vi "gamma_0__v1.vi"(10 "ƒÀ[0]":ext, 11 "ƒ¿[0]":ext) -> (3 "ƒÁ[0]":ext)   [LabVIEW 2020]
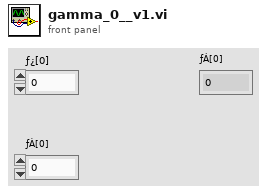
[diagram p1: front panel]
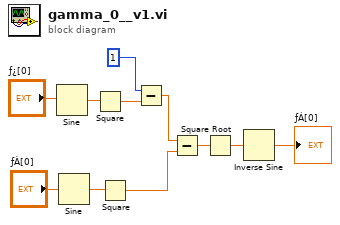
[diagram p0: block diagram]
diagram:
  n1 = Sine(x="ƒ¿[0]") -> (sin(x)=w9:ext)
  n2 = Sine(x="ƒÀ[0]") -> (sin(x)=w8:ext)
  n3 = Square(x=w9) -> (x^2=w7:ext)
  n4 = Square(x=w8) -> (x^2=w4:ext)
  n5 = Subtract(x=1, y=w7) -> (x-y=w5:ext)
  n6 = Subtract(x=w5, y=w4) -> (x-y=w3:ext)
  n7 = Square Root(x=w3) -> (sqrt(x)=w2:ext)
  n8 = Inverse Sine(1:w2) -> (0:→"ƒÁ[0]":ext)
